vi "Write Test Group Data.vi"(8 "error in (no error)":errorcluster, 10 "Test Group Data":T1, 11 "Test Group in":refnum<class "Test Group.lvclass">) -> (0 "error out":errorcluster, 3 "Test Group out":refnum<class "Test Group.lvclass">)   [LabVIEW 2016, in "Test Group Manager.lvlib" / "Test Group.lvclass"]
uses:
  Test Group.lvclass
  Test Group.lvclass/Test Group.ctl
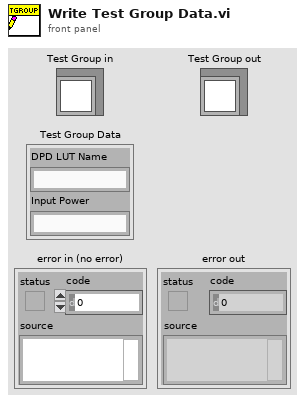
[diagram p1: front panel]
types:
  T1 = cluster{"DPD LUT Name":string, "Input Power":string}
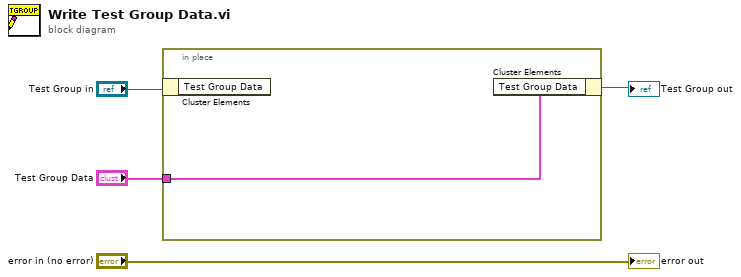
[diagram p0: block diagram]
diagram:
  n1 = in-place {
    in-place-border: "Test Group Data" -> [w5]
    n2 = in-place-cluster #1("Test Group in") -> ()  [unwired: 1 out]
    n3 = in-place-cluster #1("Test Group Data"=w5) -> (→"Test Group out":refnum<class "Test Group.lvclass">)
  }
  "error out" <- "error in (no error)"
